vi "General setup bundler-DBL.vi"(7 "Section":string, 8 "error in (no error)":errorcluster, 10 "DBL":T2, 11 "Setup.ini ref":T1) -> (0 "error out":errorcluster, 3 "Setup.ini ref":T1)   [LabVIEW 2013]
uses:
  Typedefs/Ini file interface (DBL).ctl
  <vilib>/Utility/config.llb/Config Data RefNum.ctl
  Calibration/Globals/gl_Calibration globals.vi
  Global Variables/General Globals.vi
  <vilib>/Utility/config.llb/NI_LVConfig.lvlib
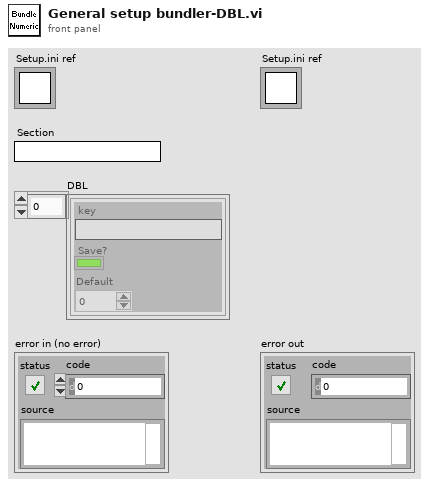
[diagram p1: front panel]
types:
  T1 = typedef "NI_LVConfig.lvlib/Config Data RefNum.ctl" = refnum<k1>
  T2 = typedef "Ini file interface (DBL).ctl" = cluster{"key":string, "Save?":bool, "Default":dbl}[]
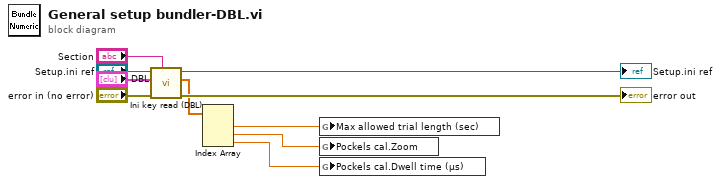
[diagram p0: block diagram]
diagram:
  n1 = call "Ini key read (DBL).vi"("Section name"="Section", "error in (no error)"="error in (no error)", "Parameter names & setup"="DBL", "Ini file refnum in"="Setup.ini ref") -> ("error out"=→"error out":errorcluster, "Value read/used"=w4:dbl[], "Ini file refnum out"=→"Setup.ini ref":T1)  [unwired: 5 in]
  n2 = Index Array(array=w4) -> (element #1=w3:dbl, element #2=w2:dbl, element #3=w1:dbl)  [unwired: 3 in]
  n3 = global write "General Globals.vi" "Max allowed trial length (sec)"(w3) -> ()
  n4 = global write "gl_Calibration globals.vi" "Pockels cal.Zoom"(w2) -> ()
  n5 = global write "gl_Calibration globals.vi" "Pockels cal.Dwell time (µs)"(w1) -> ()
